vi "ABR3-Init Stim Chans.vi"(0 "Stimulus":T29={"Ear"=enum."Left", "Waveform"=enum."TONE PIP", "Frequency (kHz)"="", "Rep rate (/sec)"=30.0, "Alternate Polarity"=FALSE, "WavFiles"="", "Level (dB SPL)"=30.0, "WavFolder"=path "", "Chirp"={"Type"=enum."AN latency-corrected", "Duration (ms)"=0.0, "Fmin (kHz)"=0.0, "Fmax (kHz)"=0.0, "precompensate"=FALSE}, "Noise"={"Seed"=0, "InvFilt"=FALSE, "AWeight"=FALSE, "afile"=path "", "Filter"={"Type"=enum."Lowpass", "CF (kHz)"=0.0, "BW (kHz)"=0.0, "Cascade"=FALSE, "Quadrature"=FALSE, "Scale Factor"=0.0, "Stages"=[], "Class"=enum."Elliptic", "Order"=0, "BWUnits"=enum."Linear"}}}, 1 "Masker":T27, 2 "Data Folder":path, 9 "Hidden":T28={"AO Samp Rate Hz"=25000.0, "Duration (ms)"=100000.0, "Ramp (ms)"=5.0, "Click width (us)"=0.5}, 11 "error in (no error)":errorcluster, 12 "Npts":i32) -> (4 "StimChans":T4[](xcontrol), 15 "error out":errorcluster)   [LabVIEW 2020]
uses:
  TypeDefs/ABR3-Stimulus.ctl
  epl-vi-lib/Utility VIs/Type Defs/Left-Right ring.ctl
  TypeDefs/ABR-Waveform Enum.ctl
  epl-vi-lib/Signal Synthesis VIs/Controls/Advanced Filter XCtl/Advanced Filter XCtl.xctl
  TypeDefs/ABR3-Hidden Params.ctl
  TypeDefs/ABR3-Masker Spec.ctl
  epl-vi-lib/Signal Synthesis VIs/Controls/Level XCtl/Level XCtl.xctl
  epl-vi-lib/Signal Synthesis VIs/Controls/Stimulus Channel (Full)/Stimulus Channel (Full).xctl
  epl-vi-lib/Signal Synthesis VIs/Controls/Multichannel (Full)/Multichannel (Full).xctl
  epl-vi-lib/Signal Synthesis VIs/Waveform VIs/Pulse Train VIs/Pulse Train Params.ctl
  epl-vi-lib/Signal Synthesis VIs/Waveform VIs/Pulse Train VIs/Pulse Polarity.ctl
  epl-vi-lib/Signal Synthesis VIs/Waveform VIs/Pulse Train VIs/PT-Continuous State.ctl
  epl-vi-lib/Signal Synthesis VIs/Controls/Level XCtl/Level Units.ctl
  epl-vi-lib/Signal Synthesis VIs/Controls/Waveform XCtl/Waveform Enum.ctl
  epl-vi-lib/Utility VIs/Type Defs/Speaker ring.ctl
panel:
  in  "Pulse Train Params":T1
  in  "Dummy":T26(xcontrol)
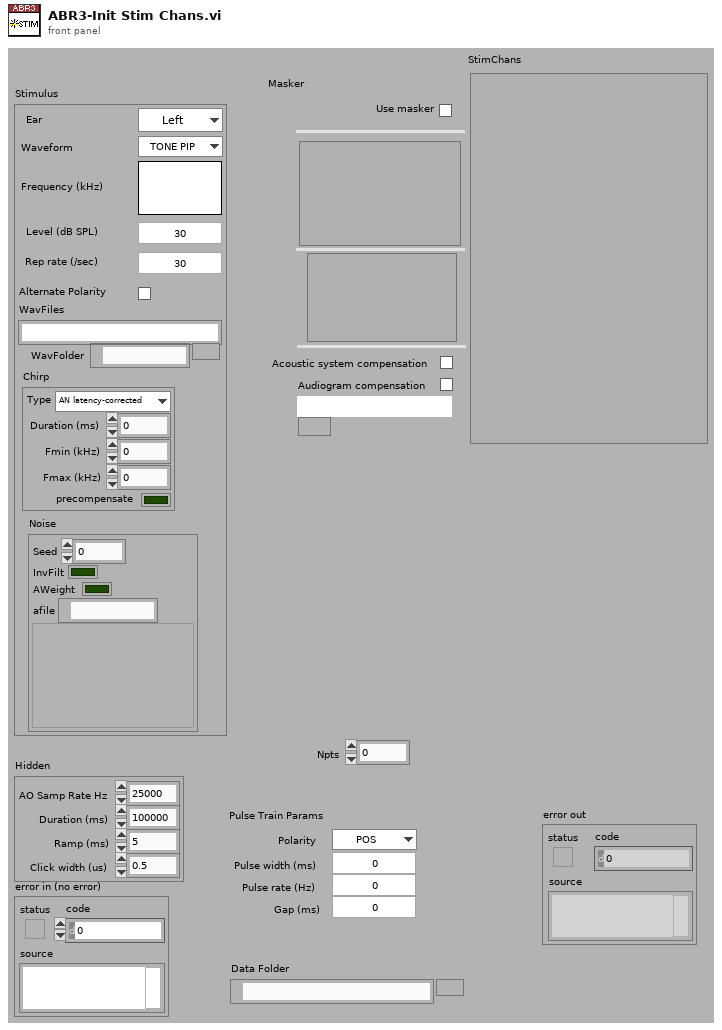
[diagram p1: front panel]
types:
  T1 = typedef "Pulse Train Params.ctl" = cluster{"Pulse width (us)":dbl, "Pulse rate (Hz)":dbl, "Gap (ms)":dbl, "Polarity":T2, "PT State":T3, "Asynch":bool}
  T2 = typedef "Pulse Polarity.ctl" = enum16{"POS", "NEG", "POS-NEG", "NEG-POS"}
  T3 = typedef "PT-Continuous State.ctl" = cluster{"Template":dbl[], "Nperiod":i32, "Index":i32, "Pulse Rate (Hz)":dbl, "Phase (cycles)":dbl, "Noff":i32}
  T4 = typedef "Stimulus Channel (Full).xctl/Full Stimulus Channel Data.ctl" = cluster{"Waveform":T5, "Filter":T19, "Burst":T21, "Level":T22, "Name":string, "Advanced":T24, "SAM":T25}
  T5 = typedef "Waveform XCtl.xctl/Waveform Data.ctl" = cluster{"Type":T6, "Tone":T7, "Pulse Train":T1, "Noise":T8, "File":T9, "FMSweep":T10, "Chirp Train":T11, "Complex Tone":cluster{"Params":T13, "Data":T15}, "Moving Ripple":T16}
  T6 = typedef "Waveform Enum.ctl" = enum16{"OFF", "Tone", "Noise", "Pulse Train", "File", "FM Sweep", "Chirp Train", "Complex Tone", "FM Tone", "Moving Ripple"}
  T7 = typedef "Tone Params.ctl" = cluster{"Frequency (kHz)":dbl, "Last Freq":dbl, "Last Phase":dbl}
  T8 = typedef "Noise Params.ctl" = cluster{"InvFilt":bool, "Noise":dbl[], "CurPt":i32, "Aweight":bool, "Seed":i32, "afile":path}
  T9 = typedef "StimFile-Params.ctl" = cluster{"Filename":path, "Signal":dbl[], "Channel":i32, "stream":bool, "offset":i32, "nreps":i32, "loops":i32, "Randomize":bool, "order":i32[], "Seed":i32, "Tokens":i32}
  T10 = typedef "FM Sweep Params.ctl" = cluster{"Rate (oct/s)":dbl, "Fmin (Hz)":dbl, "Fmax (Hz)":dbl, "Ramp (ms)":dbl, "Linear":bool}
  T11 = typedef "Chirp Train.ctl" = cluster{"Params":T12, "Data":cluster{"WF":dbl[]}}
  T12 = typedef "Chirp Train Params.ctl" = cluster{"Fmin (kHz)":dbl, "Fmax (kHz)":dbl, "Compensate":bool, "Duration (ms)":dbl}
  T13 = typedef "CT-Params.ctl" = cluster{"F0 (Hz)":dbl, "Band":cluster{"Flow (Hz)":dbl, "Fhigh (Hz)":dbl}, "Phase":T14, "Min F0 (Hz)":dbl, "Max F0 (Hz)":dbl, "ContinRandPhase":bool, "Max peak factor":dbl, "Max mod depth":dbl, "MinHarmNum":i32, "MaxHarmNum":i32, "Level Mode":enum16{"per component", "overall rms"}, "% jitter":dbl}
  T14 = typedef "CT-Phase Enum.ctl" = enum16{"Cosine", "Random", "Alternating"}
  T15 = typedef "CT-Runtime Data.ctl" = cluster{"Ncomp":i32, "MinHarm":i32, "Phase":dbl[], "Amplitude":dbl[], "Npts/frame":i32, "Last F0":dbl, "Fmin":dbl, "Fmax":dbl, "Lslope":dbl, "randphase":bool, "overall rms":bool, "fmult":dbl[], "jittered":bool}
  T16 = typedef "Moving Ripple.ctl" = cluster{"Params":T17, "Data":T18}
  T17 = typedef "Moving Ripple.Params.ctl" = cluster{"Fmin":dbl, "Fmax":dbl, "Density":dbl, "Velocity":dbl, "Depth":dbl, "Phase":dbl, "Comp/oct":i32}
  T18 = typedef "Moving Ripple.Data.ctl" = cluster{"Freq":dbl[], "A":dbl[], "phase":dbl[], "Phase":dbl}
  T19 = typedef "Advanced Filter XCtl.xctl/Filter Data.ctl" = cluster{"Type":enum16{"Lowpass", "Highpass", "Bandpass", "Bandstop", "OFF"}, "CF (kHz)":dbl, "BW (kHz)":dbl, "Cascade":bool, "Quadrature":bool, "Scale Factor":dbl, "Stages":cluster{"IIR Filter":cluster{"filter structure":enum32{"IIR 2nd Order", "IIR 4th Order"}, "Reverse Coefficients":dbl[], "Forward Coefficients":dbl[]}, "State":dbl[]}[], "Class":enum16{"Elliptic", "Butterworth"}, "Order":i32, "BWUnits":T20}
  T20 = typedef "Filter-Bandwidth Units.ctl" = enum16{"Linear", "Octaves", "Min-Max"}
  T21 = typedef "Burst Control.xctl/Burst Data.ctl" = cluster{"Active":bool, "Delay (ms)":dbl, "Duration (ms)":dbl, "Ramp (ms)":dbl, "Rate (Hz)":dbl, "Trepeat (ms)":dbl, "Repeat":bool}
  T22 = typedef "Level XCtl.xctl/Level Data.ctl" = cluster{"Level":dbl, "Units":T23, "Max":dbl, "Multiplier":dbl, "Cal File":path, "Cal":cluster{"Freq (Hz)":dbl[], "Mag (dB SPL)":dbl[], "Phase (deg)":dbl[]}}
  T23 = typedef "Level Units.ctl" = enum16{"dB atten", "dB SPL", "dB re 1 Vrms", "dB V/Hz½", "mW", "dB HL", "Volts", "dB mW"}
  T24 = typedef "Advanced Stimulus Options.xctl/Advanced Stimulus Options.ctl" = cluster{"Rep Mask":string, "AltPol":bool, "Var":string, "Expr":string, "Persist":bool}
  T25 = typedef "SAM Params.ctl" = cluster{"Active":bool, "Frequency (Hz)":dbl, "Depth":dbl, "Init Phase (cycles)":dbl, "phase (degrees)":dbl, "Asynch":bool}
  T26 = cluster{"Waveform":T5, "Filter":T19, "Burst":T21, "Level":T22, "Name":string, "Advanced":T24, "SAM":T25}
  T27 = typedef "ABR3-Masker Spec.ctl" = cluster{"Filter":cluster{"Type":enum16{"Lowpass", "Highpass", "Bandpass", "Bandstop", "OFF"}, "CF (kHz)":dbl, "BW (kHz)":dbl, "Cascade":bool, "Quadrature":bool, "Scale Factor":dbl, "Stages":cluster{"IIR Filter":cluster{"filter structure":enum32{"IIR 2nd Order", "IIR 4th Order"}, "Reverse Coefficients":dbl[], "Forward Coefficients":dbl[]}, "State":dbl[]}[], "Class":enum16{"Elliptic", "Butterworth"}, "Order":i32, "BWUnits":T20}, "Use masker":bool, "Level":cluster{"Level":dbl, "Units":T23, "Max":dbl, "Multiplier":dbl, "Cal File":path, "Cal":cluster{"Freq (Hz)":dbl[], "Mag (dB SPL)":dbl[], "Phase (deg)":dbl[]}}, "Audiogram Comp":bool, "Audiogram File":path, "InvFilt":bool}
  T28 = typedef "ABR3-Hidden Params.ctl" = cluster{"AO Samp Rate Hz":dbl, "Duration (ms)":dbl, "Ramp (ms)":dbl, "Click width (us)":dbl}
  T29 = typedef "ABR3-Stimulus.ctl" = cluster{"Ear":T30, "Waveform":T31, "Frequency (kHz)":string, "Rep rate (/sec)":dbl, "Alternate Polarity":bool, "WavFiles":string, "Level (dB SPL)":dbl, "WavFolder":path, "Chirp":cluster{"Type":enum16{"AN latency-corrected", "Arbitrary"}, "Duration (ms)":dbl, "Fmin (kHz)":dbl, "Fmax (kHz)":dbl, "precompensate":bool}, "Noise":cluster{"Seed":i32, "InvFilt":bool, "AWeight":bool, "afile":path, "Filter":cluster{"Type":enum16{"Lowpass", "Highpass", "Bandpass", "Bandstop", "OFF"}, "CF (kHz)":dbl, "BW (kHz)":dbl, "Cascade":bool, "Quadrature":bool, "Scale Factor":dbl, "Stages":cluster{"IIR Filter":cluster{"filter structure":enum32{"IIR 2nd Order", "IIR 4th Order"}, "Reverse Coefficients":dbl[], "Forward Coefficients":dbl[]}, "State":dbl[]}[], "Class":enum16{"Elliptic", "Butterworth"}, "Order":i32, "BWUnits":T20}}}
  T30 = typedef "Left-Right ring.ctl" = enum16{"Right", "Left"}
  T31 = typedef "ABR-Waveform Enum.ctl" = enum16{"TONE PIP", "CLICK", "FILE", "CHIRP", "NOISE", "VERHULST"}
  T32 = typedef "Speaker ring.ctl" = enum16{"Right primary", "Right secondary", "Left primary", "Left secondary"}
  T33 = enum16{"Lowpass", "Highpass", "Bandpass", "Bandstop", "OFF"}
  T34 = cluster{"Seed":i32, "InvFilt":bool, "AWeight":bool, "afile":path, "Filter":cluster{"Type":enum16{"Lowpass", "Highpass", "Bandpass", "Bandstop", "OFF"}, "CF (kHz)":dbl, "BW (kHz)":dbl, "Cascade":bool, "Quadrature":bool, "Scale Factor":dbl, "Stages":cluster{"IIR Filter":cluster{"filter structure":enum32{"IIR 2nd Order", "IIR 4th Order"}, "Reverse Coefficients":dbl[], "Forward Coefficients":dbl[]}, "State":dbl[]}[], "Class":enum16{"Elliptic", "Butterworth"}, "Order":i32, "BWUnits":T20}}
  T35 = cluster{"Type":enum16{"Lowpass", "Highpass", "Bandpass", "Bandstop", "OFF"}, "CF (kHz)":dbl, "BW (kHz)":dbl, "Cascade":bool, "Quadrature":bool, "Scale Factor":dbl, "Stages":cluster{"IIR Filter":cluster{"filter structure":enum32{"IIR 2nd Order", "IIR 4th Order"}, "Reverse Coefficients":dbl[], "Forward Coefficients":dbl[]}, "State":dbl[]}[], "Class":enum16{"Elliptic", "Butterworth"}, "Order":i32, "BWUnits":T20}
  T36 = cluster{"Level":dbl, "Units":T23, "Max":dbl, "Multiplier":dbl, "Cal File":path, "Cal":cluster{"Freq (Hz)":dbl[], "Mag (dB SPL)":dbl[], "Phase (deg)":dbl[]}}
  T37 = cluster{"Waveform":T5, "Filter":T19, "Burst":T21, "Level":T22, "Name":string, "Advanced":T24, "SAM":T25}[]
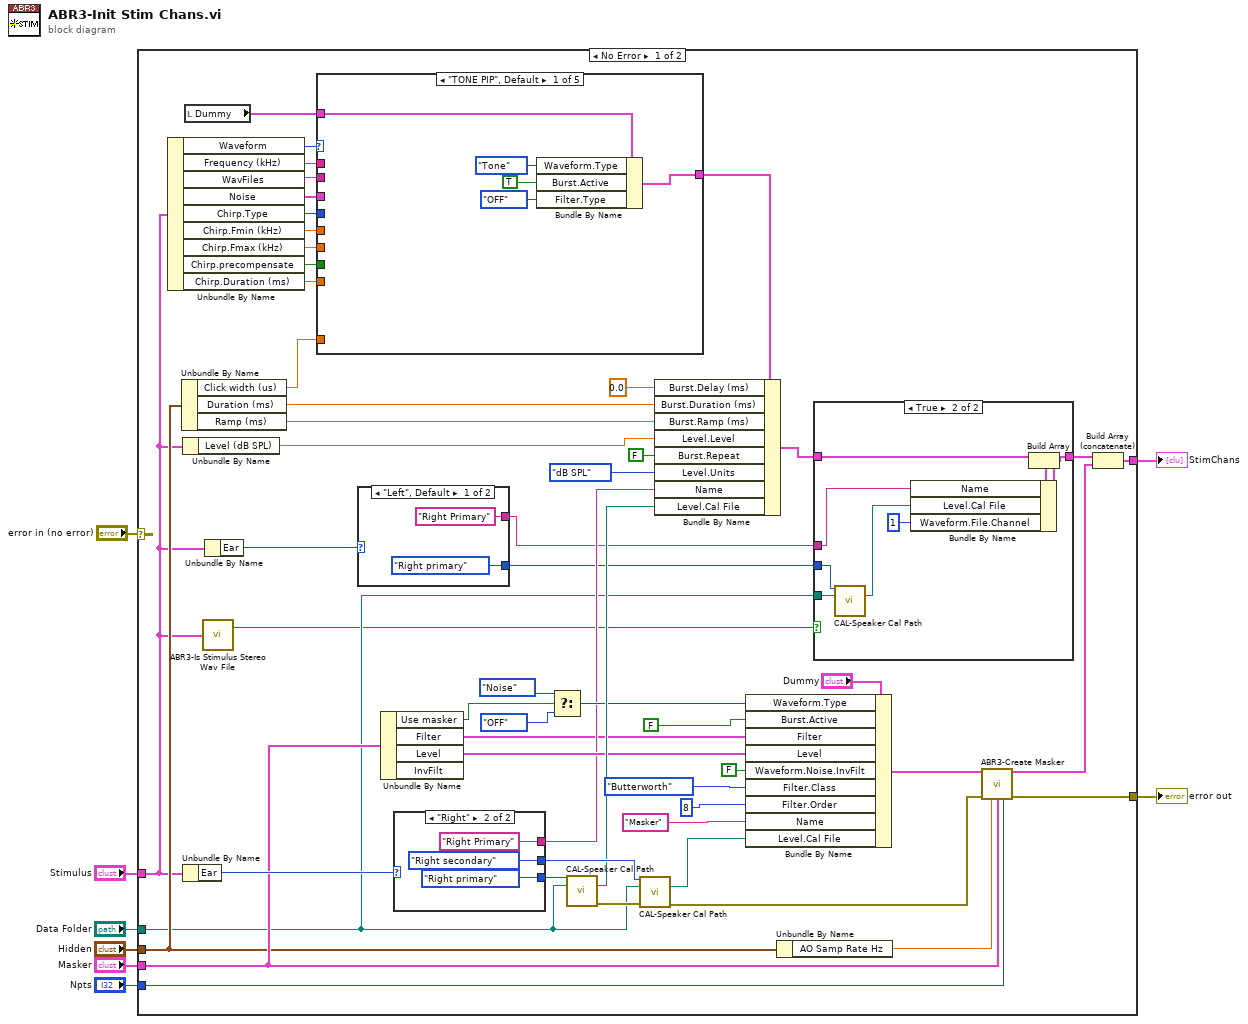
[diagram p0: block diagram]
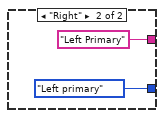
[diagram p2: hidden frame]
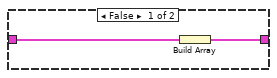
[diagram p3: hidden frame]
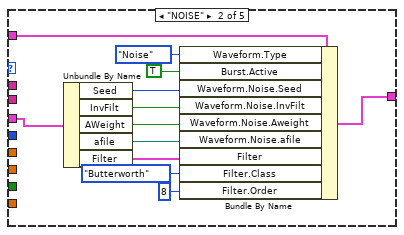
[diagram p4: hidden frame]
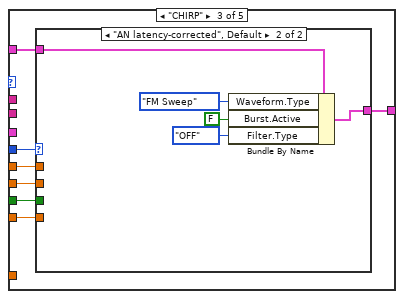
[diagram p5: hidden frame]
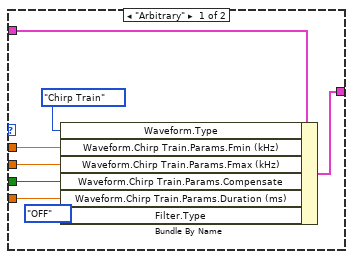
[diagram p6: hidden frame]
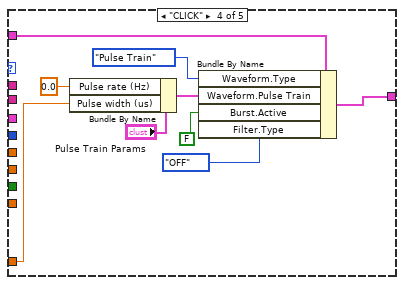
[diagram p7: hidden frame]
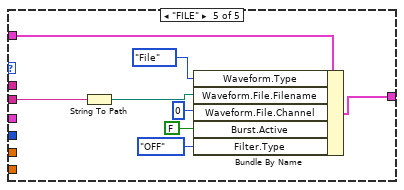
[diagram p8: hidden frame]
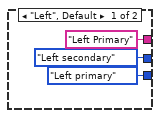
[diagram p9: hidden frame]
diagram:
  n1 = case shown="No Error" "error in (no error)" {
    selector: "error in (no error)" -> [_ w137]
    tunnel: "Hidden" -> [w28 _]
    tunnel: [w55 _] -> w7
    tunnel: "Stimulus" -> [w18 _]
    tunnel: "Data Folder" -> [w22 _]
    tunnel: [w31 w137] -> w3
    tunnel: "Masker" -> [w29 _]
    tunnel: "Npts" -> [w9 _]
    frame No Error {
      n2 = Unbundle By Name(w18) -> ("Waveform"=w42:T31, "Frequency (kHz)"=w41:string, "WavFiles"=w40:string, "Noise"=w16:T34, "Chirp.Type"=w15:enum16{"AN latency-corrected", "Arbitrary"}, "Chirp.Fmin (kHz)"=w14:dbl, "Chirp.Fmax (kHz)"=w13:dbl, "Chirp.precompensate"=w12:bool, "Chirp.Duration (ms)"=w11:dbl)
      n3 = Unbundle By Name(w28) -> ("Click width (us)"=w44:dbl, "Duration (ms)"=w61:dbl, "Ramp (ms)"=w60:dbl)
      n4 = Unbundle By Name(w18) -> ("Level (dB SPL)"=w33:dbl)
      n5 = Unbundle By Name(w18) -> ("Ear"=w51:T30)
      n6 = local read "Dummy"() -> (w45:T26)
      n7 = call "ABR3-Is Stimulus Stereo Wav File.vi"("Stimulus"=w18) -> ("Is Stereo Wav File"=w17:bool)  [unwired: 1 out]
      n8 = Unbundle By Name(w18) -> ("Ear"=w21:T30)
      n9 = case shown="\"TONE PIP\", Default" w42 {
        tunnel: w45 -> [w81 w93 w100 w120 w130]
        tunnel: w44 -> [_ _ _ w117 _]
        tunnel: [w80 w92 w99 w116 w128] -> w43
        tunnel: w41 -> [_ _ _ _ _]
        tunnel: w40 -> [_ _ _ _ w126]
        tunnel: w16 -> [_ w87 _ _ _]
        tunnel: w15 -> [_ _ w98 _ _]
        tunnel: w14 -> [_ _ w97 _ _]
        tunnel: w13 -> [_ _ w96 _ _]
        tunnel: w12 -> [_ _ w95 _ _]
        tunnel: w11 -> [_ _ w94 _ _]
        frame "TONE PIP", Default {
          n10 = Bundle By Name(cluster=w81, "Waveform.Type"=Waveform_Enum."Tone", "Burst.Active"=TRUE, "Filter.Type"=T33."OFF") -> (w80:T26)
        }
        frame "NOISE" {
          n11 = Unbundle By Name(w87) -> ("Seed"=w86:i32, "InvFilt"=w85:bool, "AWeight"=w84:bool, "afile"=w83:path, "Filter"=w82:T35)
          n12 = Bundle By Name(cluster=w93, "Waveform.Type"=Waveform_Enum."Noise", "Burst.Active"=TRUE, "Waveform.Noise.Seed"=w86, "Waveform.Noise.InvFilt"=w85, "Waveform.Noise.Aweight"=w84, "Waveform.Noise.afile"=w83, "Filter"=w82, "Filter.Class"=enum16{"Elliptic", "Butterworth"}."Butterworth", "Filter.Order"=8) -> (w92:T26)
        }
        frame "CHIRP" {
          n13 = case shown="\"AN latency-corrected\", Default" w98 {
            tunnel: w100 -> [w108 w113]
            tunnel: [w107 w112] -> w99
            tunnel: w97 -> [w105 _]
            tunnel: w96 -> [w104 _]
            tunnel: w95 -> [w103 _]
            tunnel: w94 -> [w102 _]
            frame "Arbitrary" {
              n14 = Bundle By Name(cluster=w108, "Waveform.Type"=Waveform_Enum."Chirp Train", "Waveform.Chirp Train.Params.Fmin (kHz)"=w105, "Waveform.Chirp Train.Params.Fmax (kHz)"=w104, "Waveform.Chirp Train.Params.Compensate"=w103, "Waveform.Chirp Train.Params.Duration (ms)"=w102, "Filter.Type"=T33."OFF") -> (w107:T26)
            }
            frame "AN latency-corrected", Default {
              n15 = Bundle By Name(cluster=w113, "Waveform.Type"=Waveform_Enum."FM Sweep", "Burst.Active"=FALSE, "Filter.Type"=T33."OFF") -> (w112:T26)
            }
          }
        }
        frame "CLICK" {
          n16 = Bundle By Name(cluster="Pulse Train Params", "Pulse rate (Hz)"=0.0, "Pulse width (us)"=w117) -> (w119:T1)
          n17 = Bundle By Name(cluster=w120, "Waveform.Type"=Waveform_Enum."Pulse Train", "Waveform.Pulse Train"=w119, "Burst.Active"=FALSE, "Filter.Type"=T33."OFF") -> (w116:T26)
        }
        frame "FILE" {
          n18 = String To Path(string=w126) -> (path=w125:path)
          n19 = Bundle By Name(cluster=w130, "Waveform.Type"=Waveform_Enum."File", "Waveform.File.Filename"=w125, "Waveform.File.Channel"=0, "Burst.Active"=FALSE, "Filter.Type"=T33."OFF") -> (w128:T26)
        }
      }
      n20 = case shown="\"Left\", Default" w21 {
        tunnel: [Speaker_ring."Right primary" ("Speaker") Speaker_ring."Left primary" ("Speaker")] -> w19
        tunnel: ["Right Primary" ("Name") "Left Primary" ("Name")] -> w20
        frame "Left", Default {
        }
        frame "Right" {
        }
      }
      n21 = Unbundle By Name(w29) -> ("Use masker"=w49:bool, "Filter"=w10:T35, "Level"=w37:T36)  [unwired: 1 out]
      n22 = case shown="\"Right\"" w51 {
        tunnel: [Speaker_ring."Left primary" ("Speaker") Speaker_ring."Right primary" ("Speaker")] -> w54
        tunnel: [Speaker_ring."Left secondary" ("Speaker") Speaker_ring."Right secondary" ("Speaker")] -> w53
        tunnel: ["Left Primary" ("Name") "Right Primary" ("Name")] -> w34
        frame "Left", Default {
        }
        frame "Right" {
        }
      }
      n23 = Select(t=Waveform_Enum."Noise", s=w49, f=Waveform_Enum."OFF" ("Waveform.Type")) -> (s? t:f=w47:T6)
      n24 = call "CAL-Speaker Cal Path.vi"("Speaker"=w54, "Data Folder"=w22) -> ("Cal Path"=w50:path, "error out"=w52:errorcluster)  [unwired: 12 in]
      n25 = call "CAL-Speaker Cal Path.vi"("Speaker"=w53, "Data Folder"=w22, "error in (no error)"=w52) -> ("Cal Path"=w36:path, "error out"=w32:errorcluster)  [unwired: 11 in]
      n26 = Bundle By Name(cluster=w43, "Burst.Delay (ms)"=0.0, "Burst.Duration (ms)"=w61, "Burst.Ramp (ms)"=w60, "Level.Level"=w33, "Burst.Repeat"=FALSE, "Level.Units"=Level_Units."dB SPL" ("Level.Mode"), "Name"=w34, "Level.Cal File"=w50) -> (w23:T26)
      n27 = Bundle By Name(cluster="Dummy", "Waveform.Type"=w47, "Burst.Active"=FALSE, "Filter"=w10, "Level"=w37, "Waveform.Noise.InvFilt"=FALSE, "Filter.Class"=enum16{"Elliptic", "Butterworth"}."Butterworth", "Filter.Order"=8, "Name"="Masker", "Level.Cal File"=w36) -> (w30:T26)
      n28 = Unbundle By Name(w28) -> ("AO Samp Rate Hz"=w27:dbl)
      n29 = case shown="True" w17 {
        tunnel: [w67 w76] -> w24
        tunnel: w23 -> [w68 w75]
        tunnel: w22 -> [_ w73]
        tunnel: w20 -> [_ w72]
        tunnel: w19 -> [_ w71]
        frame False {
          n30 = Build Array(w68) -> (w67:T37)
        }
        frame True {
          n31 = call "CAL-Speaker Cal Path.vi"("Speaker"=w71, "Data Folder"=w73) -> ("Cal Path"=w70:path)  [unwired: 12 in, 1 out]
          n32 = Bundle By Name(cluster=w75, "Name"=w72, "Level.Cal File"=w70, "Waveform.File.Channel"=1) -> (w74:T26)
          n33 = Build Array(w75, w74) -> (w76:T37)
        }
      }
      n34 = call "ABR3-Create Masker.vi"("StimChan"=w30, "error in (no error)"=w32, "Sampling rate (Hz)"=w27, "Masker"=w29, "Npts"=w9) -> ("Stimulus Channel out"=w26:T4, "error out"=w31:errorcluster)  [unwired: 9 in]
      n35 = Build Array (concatenate)(w24, w26) -> (w55:T4[])
    }
    frame Error {
    }
  }
  "error out" <- w3
  "StimChans" <- w7
